vi "CleanUp.vi"(0 "object in":refnum<class "Hamamatsu.lvclass">, 5 "error in (no error)":errorcluster) -> (14 "object out":refnum<class "Hamamatsu.lvclass">, 19 "error out":errorcluster)   [LabVIEW 2019, in "Hamamatsu.lvclass"]
uses:
  Hamamatsu.lvclass
  Hamamatsu.lvclass/Hamamatsu.ctl
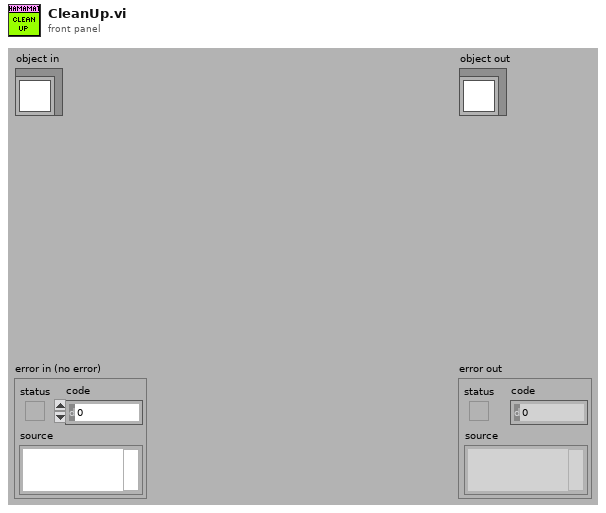
[diagram p1: front panel]
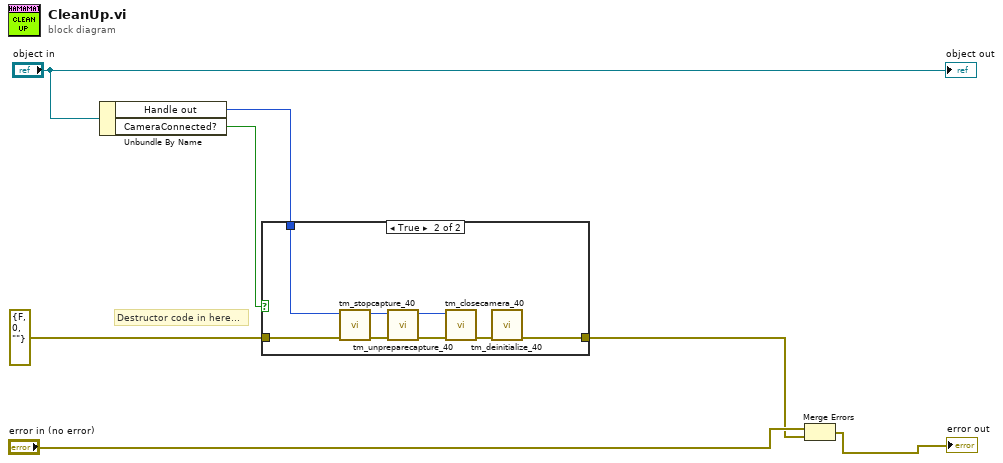
[diagram p0: block diagram]
diagram:
  # "Destructor code in here..."
  n1 = Unbundle By Name("object in") -> ("Handle out"=w4:u32, "CameraConnected?"=w1:bool)
  n2 = case shown="True" w1 {
    tunnel: w4 -> [_ w9]
    tunnel: errorcluster {"status"=FALSE, "code"=0, "source"=""} ("error in (no error)") -> [w8 w11]
    tunnel: [w8 w15] -> w2
    frame False {
    }
    frame True {
      n3 = call <userlib>:"tm_stopcapture_40.vi"("error in (no error)"=w11, "Handle in"=w9) -> ("error out"=w13:errorcluster, "Handle out"=w14:u32)  [unwired: 8 in]
      n4 = call <userlib>:"tm_unpreparecapture_40.vi"("error in (no error)"=w13, "Handle in"=w14) -> ("error out"=w12:errorcluster, "Handle out"=w10:u32)  [unwired: 8 in]
      n5 = call <userlib>:"tm_closecamera_40.vi"("error in (no error)"=w12, "Handle in"=w10) -> ("error out"=w16:errorcluster)  [unwired: 9 in]
      n6 = call <userlib>:"tm_deinitialize_40.vi"("error in (no error)"=w16) -> ("error out"=w15:errorcluster)  [unwired: 10 in]
    }
  }
  n7 = Merge Errors("error in (no error)", w2) -> (→"error out":errorcluster)
  "object out" <- "object in"
